vi "Pointer Sized Ref to Python Object Reference.vi"(1 "Py Object in":u64) -> (0 "Refnum out":T1)   [LabVIEW 2020, in "G-Embedded-Python-Interpreter-Toolkit.lvlib"]
uses:
  G-Embedded-Python-Interpreter-Toolkit.lvlib
  Python Object Type.ctl
  Python Object Reference.ctl
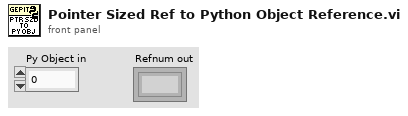
[diagram p1: front panel]
types:
  T1 = typedef "G-Embedded-Python-Interpreter-Toolkit.lvlib/Python Object Reference.ctl" = refnum<k1>
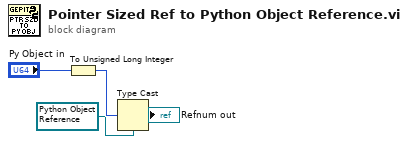
[diagram p0: block diagram]
diagram:
  w3 = T1 refnum items=["PObj"] ("Py Object")
  n1 = To Unsigned Long Integer(number="Py Object in") -> (unsigned 32bit integer=w4:u32)
  n2 = Type Cast(type=w3, x=w4) -> (*(type *) &x=→"Refnum out":T1)
